vi "MeasureDistanceInImage.vi"() -> ()   [LabVIEW 2016]
uses:
  <vilib>/vision/NI_Vision_Development_Module.lvlib
  <vilib>/Utility/inputDevices.llb/mouseAcquire.vi
panel:
  in  "Pitch":dbl=75.5
  in  "Npixels":dbl=956.746
  in  "Nstrips":dbl=42.0
  out "Length (um)":dbl
  out "Conversion: \n1 pixel to um":dbl=0.52
  out "Length (Pixels)":dbl
  out "Position 2":cluster{"X2 Value":dbl, "Y2 Value":dbl}
  in  "Set Position 2":bool
  out "Position 1":cluster{"X1 Value":dbl, "Y1 Value":dbl}
  in  "Set Position 1":bool
  out "Analysis Image":T1(plugin-control)
  out "error out":errorcluster
  in  "X coord":dbl(slide) max=2592.0 scale=0.0..2592.0
  in  "Y coord":dbl(slide) max=1944.0
  out "axis info":T2
  out "Array":T3(array[cluster])
  out "Intensity Histogram":T4(graph)
  in  "Path":path=path "C:/Users/sciollalab/Documents/TestImages/Calibration/Szoom1.png"
  # "Measure a distance in an image"
  # "Supply data for calibration calculation"
  # "readoutstrips_2 : 42, 956.746, 75.5\nSzoom1 : 16, 2323, 75.5"
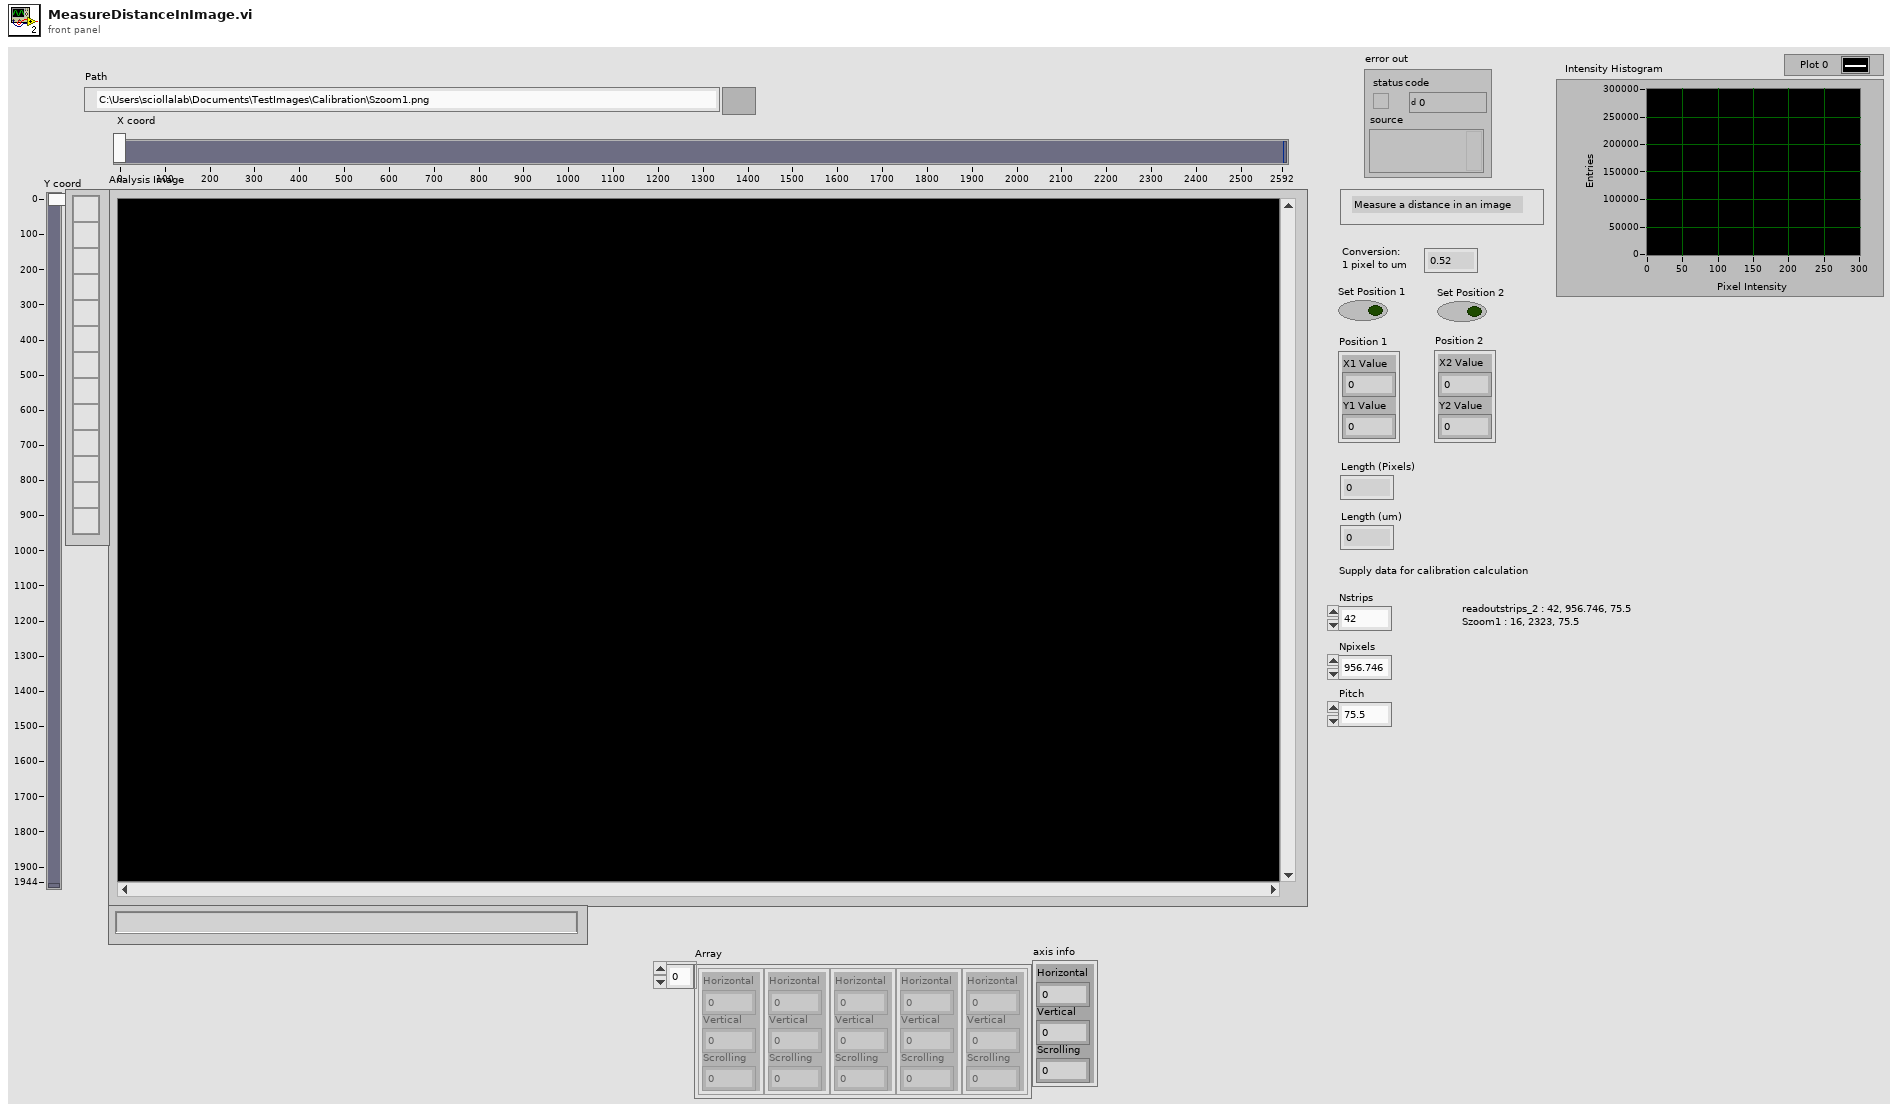
[diagram p1: front panel]
types:
  T1 = typedef "IMAQ Image.ctl" = refnum<image>
  T2 = cluster{"Horizontal":i32, "Vertical":i32, "Scrolling":i32}
  T3 = cluster{"Horizontal":i32, "Vertical":i32, "Scrolling":i32}[]
  T4 = cluster{"Starting Value":sgl, "Incremental Value":sgl, "Histogram":u32[]}
  T5 = cluster{"button 1":bool, "button 2":bool, "button 3":bool, "button 4":bool}
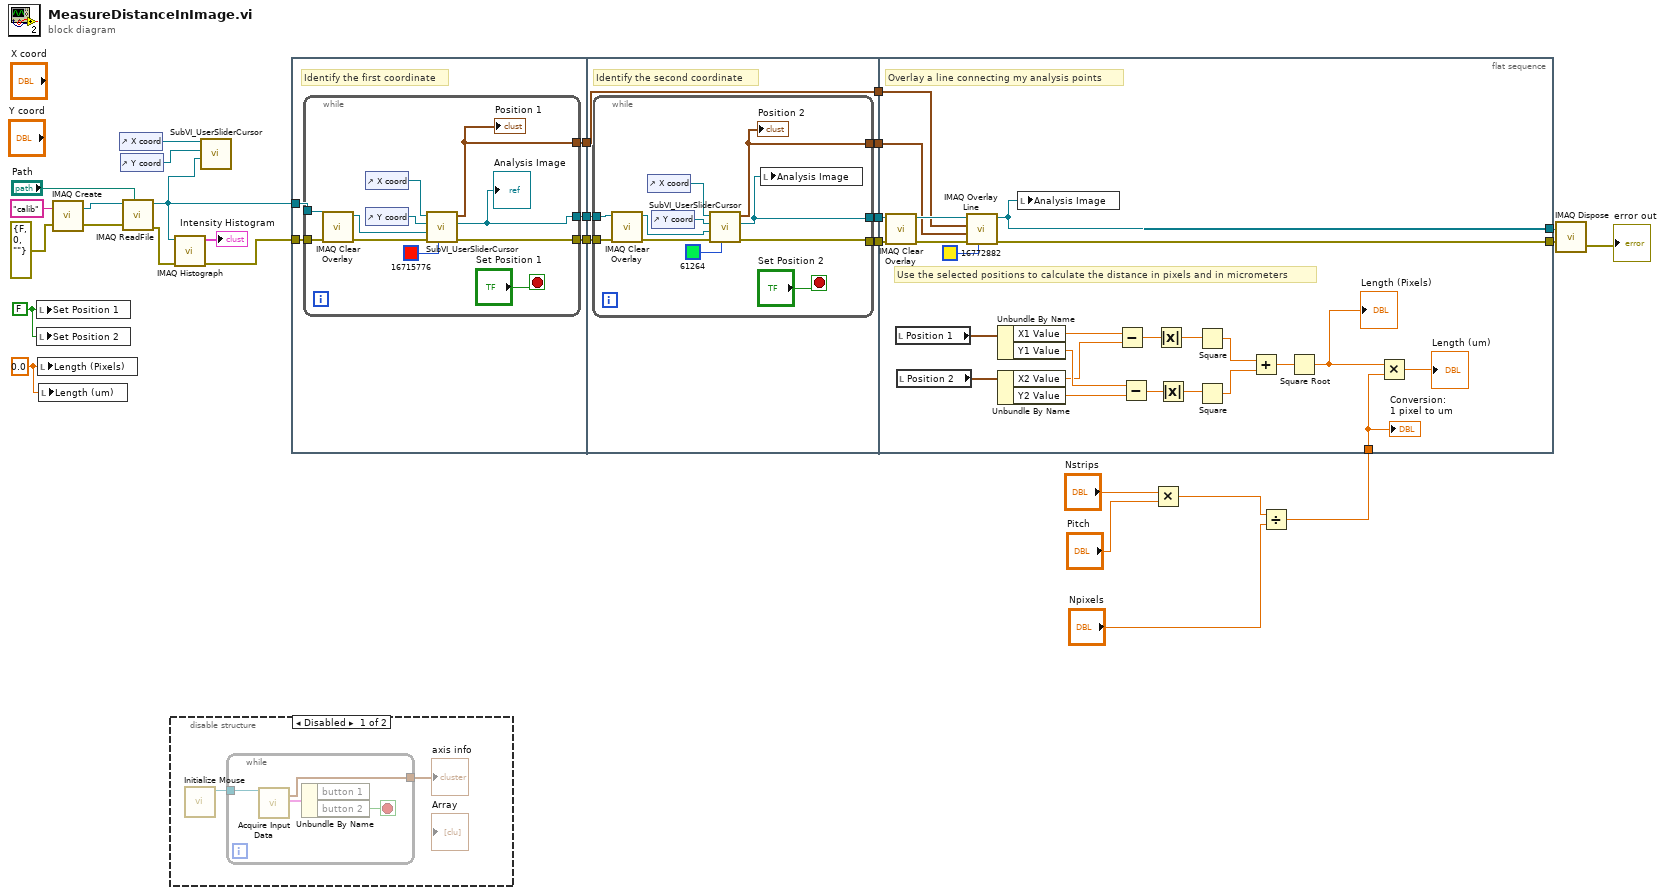
[diagram p0: block diagram]
diagram:
  w6 = 0.0 ("Length (Pixels)")
  w8 = FALSE ("Set Position 1")
  n1 = local write "Set Position 1"(w8) -> ()
  n2 = local write "Set Position 2"(w8) -> ()
  n3 = local write "Length (Pixels)"(w6) -> ()
  n4 = local write "Length (um)"(w6) -> ()
  n5 = call "IMAQ Create"("Image Name"="calib", "error in (no error)"=errorcluster {"status"=FALSE, "code"=0, "source"=""}) -> ("New Image"=w26:T1, "error out"=w25:errorcluster)  [unwired: 3 in]
  n6 = control-ref of="X coord"() -> (w19:refnum<vi>)
  n7 = control-ref of="Y coord"() -> (w18:refnum<vi>)
  n8 = call "IMAQ ReadFile"("File Path"="Path", "error in (no error)"=w25, "Image"=w26) -> ("error out"=w22:errorcluster, "Image Out"=w17:T1)  [unwired: 4 in, 3 out]
  n9 = disable-structure shown="Disabled" {
    frame Disabled {
      n10 = call <vilib>:"Initialize Mouse.vi"() -> ("device ID"=w30:refnum<k1>)  [unwired: 10 in, 1 out]
      n11 = while {
        tunnel: w30 -> [w32]
        tunnel: [w31] -> w29
        stop <- w34 stop-if-true
        n12 = call-poly <vilib>:"Acquire Input Data.vi"("device ID"=w32) -> ("axis info"=w31:T2, "button info"=w33:T5)  [unwired: 15 in, 2 out]
        n13 = Unbundle By Name(w33) -> ("button 2"=w34:bool)  [unwired: 1 out]
      }
      "axis info" <- w29
    }
    frame Enabled {
    }
  }
  n14 = call "IMAQ Histograph"("error in (no error)"=w22, "Image"=w17) -> ("error out"=w21:errorcluster, "Histogram Graph"=→"Intensity Histogram":T4)  [unwired: 6 in, 2 out]
  n15 = call "SubVI_UserSliderCursor.vi"("X slider refnum in"=w19, "Y slider refnum in"=w18, "Image RefNum"=w17) -> ()  [unwired: 7 in]
  n16 = flat-sequence {
    tunnel: w21 -> [w39]
    tunnel: w17 -> [w36]
    tunnel: [w38] -> w16
    tunnel: [w37] -> w15
    tunnel: [w35] -> w14
    tunnel: w16 -> [w55]
    tunnel: w15 -> [w54]
    tunnel: w14 -> [w53]
    tunnel: [w56] -> w13
    tunnel: [w53] -> w12
    tunnel: [w52] -> w11
    tunnel: [w51] -> w7
    tunnel: w13 -> [w85]
    tunnel: w12 -> [w84]
    tunnel: w11 -> [w92]
    tunnel: [w89] -> w10
    tunnel: [w88] -> w9
    tunnel: w7 -> [w86]
    tunnel: w1 -> [w68]
    frame #0 {
      # "Identify the first coordinate"
      n17 = while {
        tunnel: w36 -> [w50]
        tunnel: w39 -> [w49]
        tunnel: [w41] -> w38
        tunnel: [w42] -> w37
        tunnel: [w40] -> w35
        stop <- "Set Position 1" stop-if-true
        n18 = call "IMAQ Clear Overlay"("error in (no error)"=w49, "Image"=w50) -> ("error out"=w46:errorcluster, "Image Out"=w45:T1)  [unwired: 8 in]
        n19 = control-ref of="X coord"() -> (w43:refnum<vi>)
        n20 = control-ref of="Y coord"() -> (w44:refnum<vi>)
        n21 = call "SubVI_UserSliderCursor.vi"("Axes colour"=u32 16715776, "error in (no error)"=w46, "Image RefNum In"=w45, "Y slider refnum"=w44, "X slider refnum"=w43) -> ("error out"=w42:errorcluster, "Image Refnum out"=w41:T1, "Cross Point"=w40:cluster{"X coordinate":dbl, "Y coordinate":dbl})  [unwired: 4 in]
        "Analysis Image" <- w41
        "Position 1" <- w40
      }
    }
    frame #1 {
      # "Identify the second coordinate"
      n22 = while {
        tunnel: [w66] -> w52
        tunnel: [w57] -> w56
        tunnel: w55 -> [w63]
        tunnel: w54 -> [w62]
        tunnel: [w59] -> w51
        stop <- "Set Position 2" stop-if-true
        n23 = call "IMAQ Clear Overlay"("error in (no error)"=w62, "Image"=w63) -> ("error out"=w67:errorcluster, "Image Out"=w58:T1)  [unwired: 8 in]
        n24 = control-ref of="X coord"() -> (w60:refnum<vi>)
        n25 = control-ref of="Y coord"() -> (w61:refnum<vi>)
        n26 = call "SubVI_UserSliderCursor.vi"("Axes colour"=u32 61264, "error in (no error)"=w67, "Image RefNum In"=w58, "Y slider refnum"=w61, "X slider refnum"=w60) -> ("error out"=w66:errorcluster, "Image Refnum out"=w59:T1, "Cross Point"=w57:cluster{"X coordinate":dbl, "Y coordinate":dbl})  [unwired: 4 in]
        "Position 2" <- w57
        n27 = local write "Analysis Image"(w59) -> ()
      }
    }
    frame #2 {
      # "Use the selected positions to calculate the distance in pixels and in micrometers"
      # "Overlay a line connecting my analysis points"
      n28 = call "IMAQ Clear Overlay"("error in (no error)"=w92, "Image"=w86) -> ("error out"=w90:errorcluster, "Image Out"=w91:T1)  [unwired: 8 in]
      n29 = local read "Position 1"() -> (w72:cluster{"X1 Value":dbl, "Y1 Value":dbl})
      n30 = local read "Position 2"() -> (w73:cluster{"X2 Value":dbl, "Y2 Value":dbl})
      n31 = call "IMAQ Overlay Line"("Color"=u32 16772882, "error in (no error)"=w90, "End Point"=w85, "Start Point"=w84, "Image"=w91) -> ("error out"=w88:errorcluster, "Image Out"=w89:T1)  [unwired: 5 in]
      n32 = Unbundle By Name(w72) -> ("X1 Value"=w74:dbl, "Y1 Value"=w76:dbl)
      n33 = Unbundle By Name(w73) -> ("X2 Value"=w75:dbl, "Y2 Value"=w77:dbl)
      n34 = local write "Analysis Image"(w89) -> ()
      n35 = Subtract(x=w74, y=w75) -> (x-y=w78:dbl)
      n36 = Subtract(x=w76, y=w77) -> (x-y=w79:dbl)
      n37 = Absolute Value(x=w78) -> (abs(x)=w80:dbl)
      n38 = Absolute Value(x=w79) -> (abs(x)=w81:dbl)
      n39 = Square(x=w80) -> (x^2=w69:dbl)
      n40 = Square(x=w81) -> (x^2=w70:dbl)
      n41 = Add(x=w69, y=w70) -> (x+y=w71:dbl)
      n42 = Square Root(x=w71) -> (sqrt(x)=w82:dbl)
      "Length (Pixels)" <- w82
      n43 = Multiply(x=w82, y=w68) -> (x*y=→"Length (um)":dbl)
      "Conversion: \n1 pixel to um" <- w68
    }
  }
  n44 = Multiply(x="Nstrips", y="Pitch") -> (x*y=w2:dbl)
  n45 = Divide(x=w2, y="Npixels") -> (x/y=w1:dbl)
  n46 = call "IMAQ Dispose"("Image"=w10, "error in (no error)"=w9) -> ("error out"=→"error out":errorcluster)  [unwired: 4 in]
